vi "GetDataEventConfig.vi"(8 "error in (no error)":errorcluster, 9 "DataGroup":string, 10 "AcqParams":variant, 11 "map in":T5) -> (0 "error out":errorcluster, 1 "OpState":string, 2 "acq params":T1, 3 "map out":T5)   [LabVIEW 2017, in "McsaDataEventCreator.lvlib"]
uses:
  <vilib>/addons/InsightCM/Devices/Shared/Mcsa/McsaDataEventCreator/McsaDataEventCreator.lvlib
  <vilib>/addons/PointValueMap/controls/PointMap.ctl
  <vilib>/addons/InsightCM/Devices/Shared/Mcsa/McsaDataEventCreator/controls/AcqParams.ctl
  <vilib>/addons/InsightCM/Devices/Shared/Common/DataAccumulator/controls/AccumulationSettings.ctl
  <vilib>/addons/InsightCM/Devices/Shared/Common/DataAccumulator/controls/accumulationType.ctl
  <vilib>/addons/InsightCM/Devices/Shared/Common/DVRBuffer/controls/BufferLocation.ctl
  <vilib>/addons/PointValueMap/subVIs/Point_Read_string.vi
  <vilib>/addons/PointValueMap/PointValueMap.lvlib
  <vilib>/addons/InsightCM/Devices/Shared/Common/DVRBuffer/DVRBuffer.lvlib
  <vilib>/addons/InsightCM/Devices/Shared/Common/DataAccumulator/DataAccumulator.lvlib
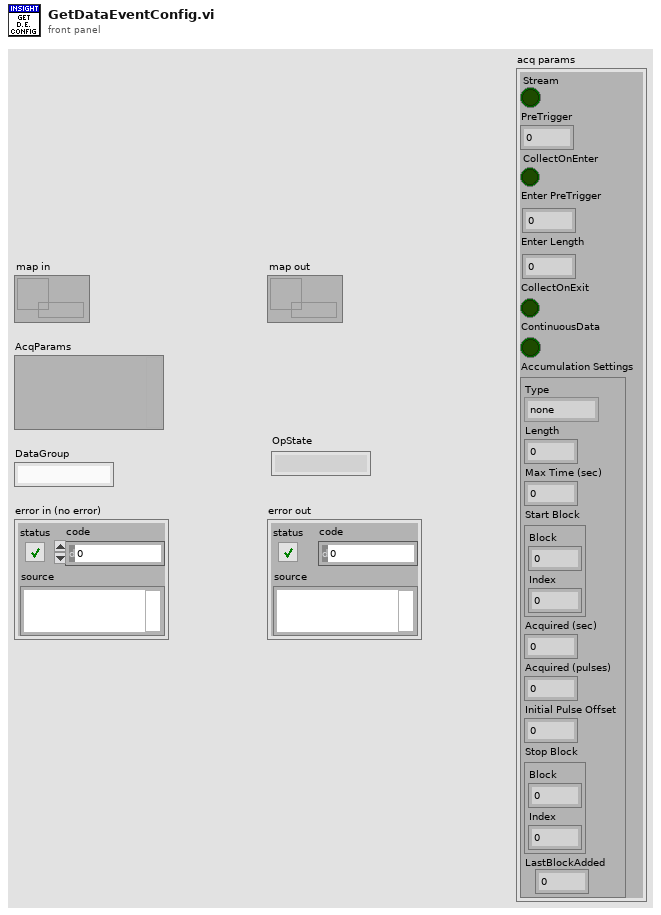
[diagram p1: front panel]
types:
  T1 = typedef "McsaDataEventCreator.lvlib/AcqParams.ctl" = cluster{"Stream":bool, "PreTrigger":i32, "CollectOnEnter":bool, "Enter PreTrigger":i32, "Enter Length":dbl, "CollectOnExit":bool, "ContinuousData":bool, "Accumulation Settings":T2}
  T2 = typedef "DataAccumulator.lvlib/AccumulationSettings.ctl" = cluster{"Type":T3, "Length":dbl, "Max Time (sec)":dbl, "Start Block":T4, "Acquired (sec)":dbl, "Acquired (pulses)":i32, "Initial Pulse Offset":dbl, "Stop Block":T4, "LastBlockAdded":u32}
  T3 = typedef "DataAccumulator.lvlib/accumulationType.ctl" = enum16{"none", "seconds", "revolutions"}
  T4 = typedef "DVRBuffer.lvlib/BufferLocation.ctl" = cluster{"Block":u32, "Index":i32}
  T5 = typedef "PointValueMap.lvlib/PointMap.ctl" = refnum<data-value>
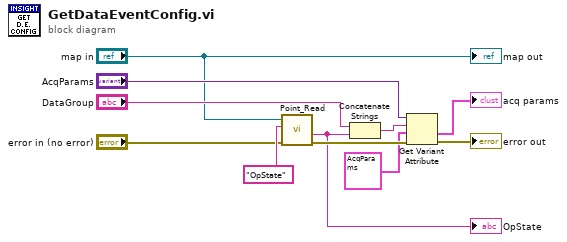
[diagram p0: block diagram]
diagram:
  n1 = call-poly <vilib>:"Point_Read.vi"("Error In"="error in (no error)", "Tag"="OpState", "Map"="map in") -> ("Error Out"=w9:errorcluster, "Value"=w1:string)  [unwired: 3 in, 4 out]
  "OpState" <- w1
  n2 = Concatenate Strings("DataGroup", w1) -> (w10:string)
  n3 = Get Variant Attribute(Variant="AcqParams", name=w10, default value (empty Variant)=T1 {"Stream"=FALSE, "PreTrigger"=0, "CollectOnEnter"=FALSE, "Enter PreTrigger"=0, "Enter Length"=0.0, "CollectOnExit"=FALSE, "ContinuousData"=FALSE, "Accumulation Settings"={"Type"=enum."none", "Length"=0.0, "Max Time (sec)"=0.0, "Start Block"={"Block"=0, "Index"=0}, "Acquired (sec)"=0.0, "Acquired (pulses)"=0, "Initial Pulse Offset"=0.0, "Stop Block"={"Block"=0, "Index"=0}, "LastBlockAdded"=0}} ("AcqParams"), error in=w9) -> (value=→"acq params":T1, error out=→"error out":errorcluster)  [unwired: 2 out]
  "map out" <- "map in"
